vi "CCD Acquire Spectrum vs Pixels.vi"(11 "error in":errorcluster) -> (15 "error out":errorcluster)   [LabVIEW 2020, in "Examples.lvlib"]
doc: "Example for a CCD spectrum acquisition."
uses:
  Examples.lvlib
  4aef6941-9f58-45d1-a797-2b486d7897ac.vi
  Classes/CCD/CCD.lvclass
  <vilib>/Utility/file.llb/Write Delimited Spreadsheet (DBL).vi
panel:
  out "XY Graph":cluster{"xAxis":dbl[], "imageData":dbl[]}(graph)
  # "Connector Pane"
  # "Locals"
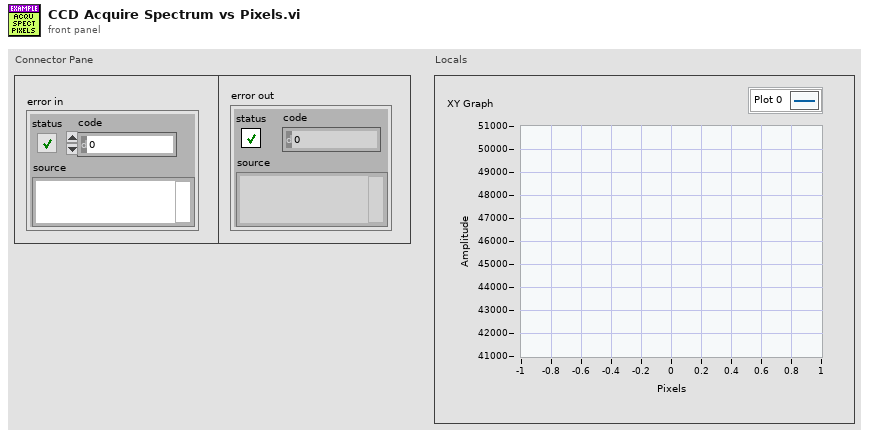
[diagram p1: front panel]
types:
  T1 = cluster{"ROI-index":i32, "xOrigin":i32, "yOrigin":i32, "xSize":i32, "ySize":i32, "xBin":i32, "yBin":i32}
  T2 = typedef "horiba.lvlib/CCD.lvclass/ccdAcquisitionData.ctl" = cluster{"acqIndex":i32, "ROIs":T3[], "timestamp":string}
  T3 = typedef "horiba.lvlib/CCD.lvclass/imageAcqData.ctl" = cluster{"roiMetaData":T4, "xAxis":dbl[], "yData":dbl[][]}
  T4 = typedef "horiba.lvlib/CCD.lvclass/roiMetaData.ctl" = cluster{"roiIndex":i32, "xBinning":i32, "xOrigin":i32, "xSize":i32, "yBinning":i32, "yOrigin":i32, "ySize":i32}
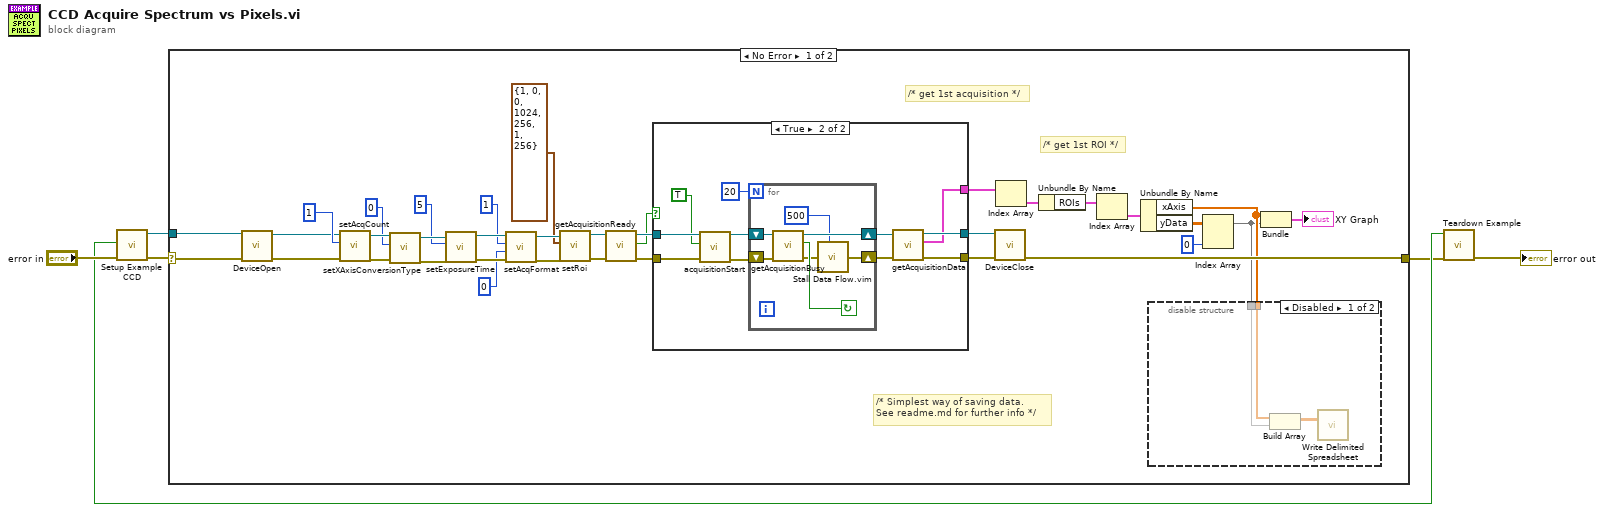
[diagram p0: block diagram]
diagram:
  n1 = call "Setup Example CCD.vi"("error in (no error)"="error in") -> ("error out"=w4:errorcluster, "Module Was Already Running?"=w2:bool, "CCD out"=w3:refnum<class "CCD.lvclass">)  [unwired: 8 in]
  n2 = case shown="No Error" w4 {
    selector: w4 -> [w41 w65]
    tunnel: w3 -> [w12 _]
    tunnel: [w21 w65] -> w1
    frame No Error {
      # "/* Simplest way of saving data.\nSee readme.md for further info */"
      # "/* get 1st ROI */"
      # "/* get 1st acquisition */"
      n3 = call-dynamic "DeviceOpen.vi"("error in (no error)"=w41, "CCD in"=w12) -> ("error out"=w13:errorcluster, "CCD out"=w11:refnum<class "CCD.lvclass">)  [unwired: 6 in, 2 out]
      n4 = call "setAcqCount.vi"("error in (no error)"=w13, "count"=1, "CCD in"=w11) -> ("error out"=w39:errorcluster, "CCD out"=w38:refnum<class "CCD.lvclass">)  [unwired: 5 in, 2 out]
      n5 = call "setXAxisConversionType.vi"("error in (no error)"=w39, "type"=0, "CCD in"=w38) -> ("error out"=w36:errorcluster, "CCD out"=w35:refnum<class "CCD.lvclass">)  [unwired: 5 in, 2 out]
      n6 = call "setExposureTime.vi"("error in (no error)"=w36, "exposure time [ms] or [us]"=5, "CCD in"=w35) -> ("error out"=w33:errorcluster, "CCD out"=w32:refnum<class "CCD.lvclass">)  [unwired: 5 in, 2 out]
      n7 = call "setAcqFormat.vi"("error in (no error)"=w33, "format"=0, "number of ROIs"=1, "CCD in"=w32) -> ("error out"=w29:errorcluster, "CCD out"=w28:refnum<class "CCD.lvclass">)  [unwired: 4 in, 2 out]
      n8 = call "setRoi.vi"("error in (no error)"=w29, "roiConfig"=T1 {"ROI-index"=1, "xOrigin"=0, "yOrigin"=0, "xSize"=1024, "ySize"=256, "xBin"=1, "yBin"=256}, "CCD in"=w28) -> ("error out"=w27:errorcluster, "CCD out"=w26:refnum<class "CCD.lvclass">)  [unwired: 5 in, 2 out]
      n9 = call "getAcquisitionReady.vi"("error in (no error)"=w27, "CCD in"=w26) -> ("error out"=w25:errorcluster, "ready"=w23:bool, "CCD out"=w24:refnum<class "CCD.lvclass">)  [unwired: 7 in]
      n10 = case shown="True" w23 {
        tunnel: w25 -> [w45 w57]
        tunnel: w24 -> [w46 w56]
        tunnel: [w45 w50] -> w22
        tunnel: [w46 w48] -> w20
        tunnel: [_ w47] -> w18
        frame False {
        }
        frame True {
          n11 = call "acquisitionStart.vi"("error in (no error)"=w57, "openShutter"=TRUE, "CCD in"=w56) -> ("error out"=w52:errorcluster, "CCD out"=w51:refnum<class "CCD.lvclass">)  [unwired: 5 in, 2 out]
          n12 = for {
            N: 20 -> [_]
            shift-right: [w60] -> w53
            shift-left: w52 -> [w63]
            shift-right: [w59] -> w49
            shift-left: w51 -> [w64]
            stop <- w62 continue-if-true
            n13 = call "getAcquisitionBusy.vi"("error in (no error)"=w63, "CCD in"=w64) -> ("error out"=w61:errorcluster, "isBusy"=w62:bool, "CCD out"=w59:refnum<class "CCD.lvclass">)  [unwired: 7 in]
            n14 = call "Stall Data Flow.vim"("value in"=w61, "milliseconds to wait"=u32 500) -> ("value out"=w60:errorcluster)  [unwired: 1 out]
          }
          n15 = call "getAcquisitionData.vi"("error in (no error)"=w53, "CCD in"=w49) -> ("error out"=w50:errorcluster, "ccdAcquisitions"=w47:T2[], "CCD out"=w48:refnum<class "CCD.lvclass">)  [unwired: 6 in, 1 out]
        }
      }
      n16 = call-dynamic "DeviceClose.vi"("error in (no error)"=w22, "CCD in"=w20) -> ("error out"=w21:errorcluster)  [unwired: 5 in, 4 out]
      n17 = Index Array(array=w18) -> (element=w17:T2)  [unwired: 1 in]
      n18 = Unbundle By Name(w17) -> ("ROIs"=w16:T3[])
      n19 = Index Array(array=w16) -> (element=w15:T3)  [unwired: 1 in]
      n20 = Unbundle By Name(w15) -> ("xAxis"=w10:dbl[], "yData"=w9:dbl[][])
      n21 = Index Array(array=w9, index (col)=0 ("disabled index (col)")) -> (element=w8:dbl[])  [unwired: 1 in]
      n22 = disable-structure shown="Disabled" {
        disable-tunnel: w10 -> [w44 _]
        disable-tunnel: w8 -> [w43 _]
        frame Disabled {
          n23 = Build Array(w44, w43) -> (w42:dbl[][])
          n24 = call-poly <vilib>:"Write Delimited Spreadsheet.vi"("2D data"=w42) -> ()  [unwired: 13 in, 2 out]
        }
        frame Enabled {
        }
      }
      n25 = Bundle("xAxis"=w10, "yData"=w8) -> (→"XY Graph":cluster{"xAxis":dbl[], "yData":dbl[]})  [unwired: 1 in]
    }
    frame Error {
    }
  }
  n26 = call "Teardown Example.vi"("error in (no error)"=w1, "Module Was Already Running?"=w2) -> ("error out"=→"error out":errorcluster)  [unwired: 9 in]
